vi "Find Button Ering.vi"(4 "Find Ering Setting":T4 {"Options"."Edge Options"."Edge Polarity" items=["All Edges", "Rising Edges", "Falling Edges"]; "Options"."Edge Options"."Minimum Edge Strength" format="%.2f"; "Options"."Edge Options"."Width" step=2; "Options"."Edge Options"."Kernel Size" step=2}, 6 "Find Center Setting":T4 {"Options"."Edge Options"."Edge Polarity" items=["All Edges", "Rising Edges", "Falling Edges"]; "Options"."Edge Options"."Minimum Edge Strength" format="%.2f"; "Options"."Edge Options"."Width" step=2; "Options"."Edge Options"."Kernel Size" step=2}, 7 "Match Position":T7, 8 "error in (no error)":errorcluster, 9 "Ering ROI":T5 {"Contours"."Type" items=["No Selection", "Point", "Line", "Rectangle", "Oval", "Polygon", "Freehand Region", "Annulus", "Unused2", "Unused3", "Broken Line", "Freehand Line", "Rotated Rectangle"]}, 10 "Center ROI":T5 {"Contours"."Type" items=["No Selection", "Point", "Line", "Rectangle", "Oval", "Polygon", "Freehand Region", "Annulus", "Unused2", "Unused3", "Broken Line", "Freehand Line", "Rotated Rectangle"]}, 11 "Image in":T6) -> (0 "error out":errorcluster, 2 "Array of Fittings":T1)   [LabVIEW 2017]
uses:
  <vilib>/vision/Measure.llb/Edge Options.ctl
  <vilib>/vision/Measure.llb/Edge Polarity.ctl
  <vilib>/vision/Image Controls.llb/IMAQ Image.ctl
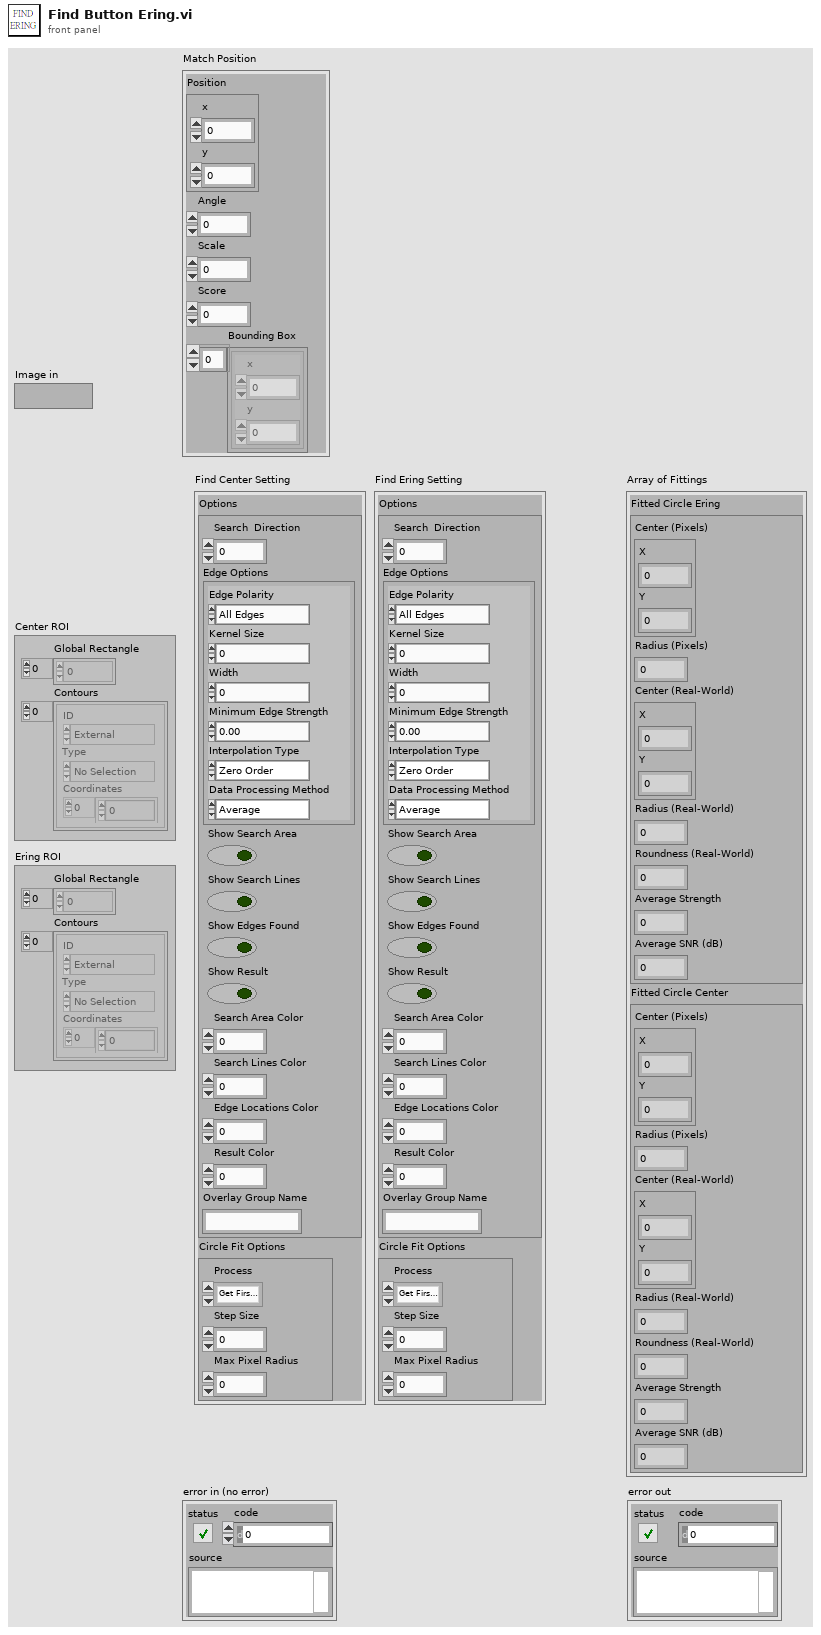
[diagram p1: front panel]
types:
  T1 = cluster{"Fitted Circle Ering":cluster{"Center (Pixels)":cluster{"X":sgl, "Y":sgl}, "Radius (Pixels)":dbl, "Center (Real-World)":cluster{"X":sgl, "Y":sgl}, "Radius (Real-World)":dbl, "Roundness (Real-World)":dbl, "Average Strength":dbl, "Average SNR (dB)":dbl}, "Fitted Circle Center":cluster{"Center (Pixels)":cluster{"X":sgl, "Y":sgl}, "Radius (Pixels)":dbl, "Center (Real-World)":cluster{"X":sgl, "Y":sgl}, "Radius (Real-World)":dbl, "Roundness (Real-World)":dbl, "Average Strength":dbl, "Average SNR (dB)":dbl}}
  T2 = typedef "Edge Options.ctl" = cluster{"Edge Polarity":T3, "Kernel Size":u32, "Width":u32, "Minimum Edge Strength":sgl, "Interpolation Type":enum32{"Zero Order", "Bilinear", "Quadratic", "Cubic", "Bilinear Fixed"}, "Data Processing Method":enum32{"Average", "Median"}}
  T3 = typedef "Edge Polarity.ctl" = u32
  T4 = cluster{"Options":cluster{"Search  Direction":u32, "Edge Options":T2, "Show Search Area":bool, "Show Search Lines":bool, "Show Edges Found":bool, "Show Result":bool, "Search Area Color":u32, "Search Lines Color":u32, "Edge Locations Color":u32, "Result Color":u32, "Overlay Group Name":string}, "Circle Fit Options":cluster{"Process":enum16{"Get First Edge", "Get First + Last Edge", "Get All Edges", "Get Best Edge"}, "Step Size":dbl, "Max Pixel Radius":i32}}
  T5 = typedef "ROI Descriptor" = cluster{"Global Rectangle":i32[], "Contours":cluster{"ID":enum32{"External", "Internal"}, "Type":u32, "Coordinates":i32[]}[]}
  T6 = typedef "IMAQ Image.ctl" = refnum<image>
  T7 = cluster{"Position":cluster{"x":sgl, "y":sgl}, "Angle":sgl, "Scale":sgl, "Score":sgl, "Bounding Box":cluster{"x":sgl, "y":sgl}[]}
  T8 = cluster{"Center (Pixels)":cluster{"X":sgl, "Y":sgl}, "Radius (Pixels)":dbl, "Center (Real-World)":cluster{"X":sgl, "Y":sgl}, "Radius (Real-World)":dbl, "Roundness (Real-World)":dbl, "Average Strength":dbl, "Average SNR (dB)":dbl}
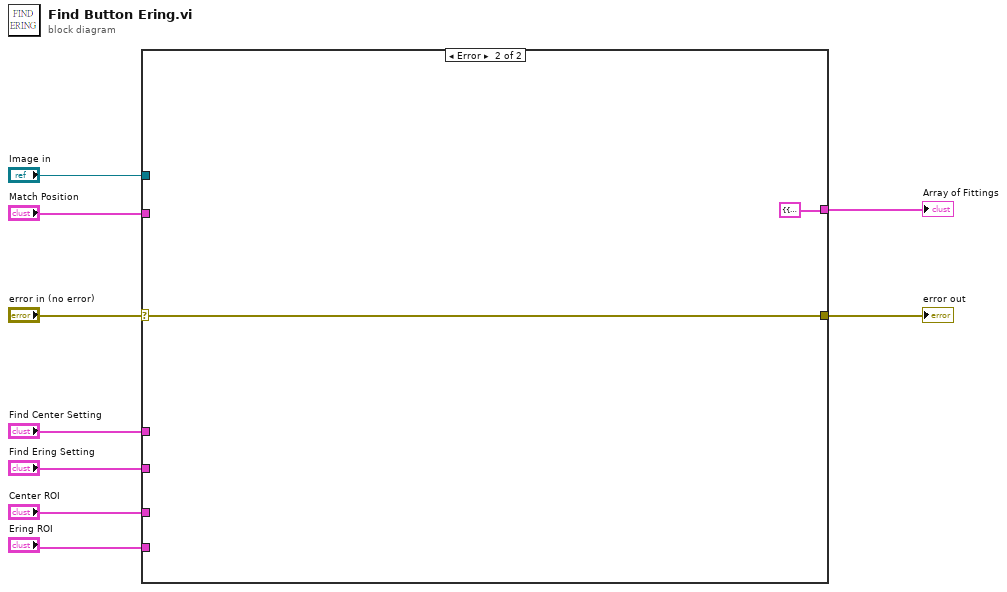
[diagram p0: block diagram]
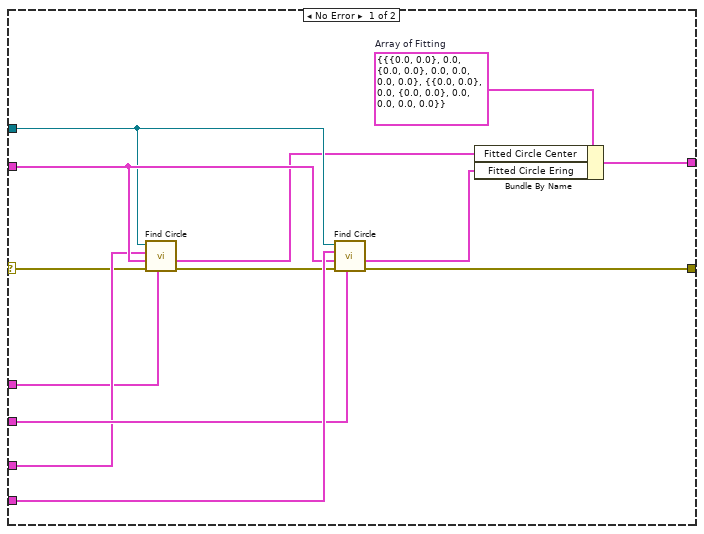
[diagram p2: hidden frame]
diagram:
  n1 = case shown="Error" "error in (no error)" {
    selector: "error in (no error)" -> [w10 w24]
    tunnel: "Ering ROI" -> [w22 _]
    tunnel: "Match Position" -> [w21 _]
    tunnel: "Find Ering Setting" -> [w19 _]
    tunnel: [w18 w24] -> w6
    tunnel: "Image in" -> [w17 _]
    tunnel: "Center ROI" -> [w16 _]
    tunnel: "Find Center Setting" -> [w15 _]
    tunnel: [w11 T1 {"Fitted Circle Ering"={"Center (Pixels)"={"X"=0.0, "Y"=0.0}, "Radius (Pixels)"=0.0, "Center (Real-World)"={"X"=0.0, "Y"=0.0}, "Radius (Real-World)"=0.0, "Roundness (Real-World)"=0.0, "Average Strength"=0.0, "Average SNR (dB)"=0.0}, "Fitted Circle Center"={"Center (Pixels)"={"X"=0.0, "Y"=0.0}, "Radius (Pixels)"=0.0, "Center (Real-World)"={"X"=0.0, "Y"=0.0}, "Radius (Real-World)"=0.0, "Roundness (Real-World)"=0.0, "Average Strength"=0.0, "Average SNR (dB)"=0.0}} ("Array of Fitting")] -> w2
    frame No Error {
      w14 = T1 {"Fitted Circle Ering"={"Center (Pixels)"={"X"=0.0, "Y"=0.0}, "Radius (Pixels)"=0.0, "Center (Real-World)"={"X"=0.0, "Y"=0.0}, "Radius (Real-World)"=0.0, "Roundness (Real-World)"=0.0, "Average Strength"=0.0, "Average SNR (dB)"=0.0}, "Fitted Circle Center"={"Center (Pixels)"={"X"=0.0, "Y"=0.0}, "Radius (Pixels)"=0.0, "Center (Real-World)"={"X"=0.0, "Y"=0.0}, "Radius (Real-World)"=0.0, "Roundness (Real-World)"=0.0, "Average Strength"=0.0, "Average SNR (dB)"=0.0}}  # Array of Fitting
      n2 = call "Find Circle.vi"("Find Circle Setting"=w15, "error in (no error)"=w10, "Matches (pixel)"=w21, "ROI Descriptor"=w16, "Image"=w17) -> ("error out"=w20:errorcluster, "Fitted Circle"=w12:T8)  [unwired: 3 in, 2 out]
      n3 = call "Find Circle.vi"("Find Circle Setting"=w19, "error in (no error)"=w20, "Matches (pixel)"=w21, "ROI Descriptor"=w22, "Image"=w17) -> ("error out"=w18:errorcluster, "Fitted Circle"=w13:T8)  [unwired: 3 in, 2 out]
      n4 = Bundle By Name(cluster=w14, "Fitted Circle Center"=w12, "Fitted Circle Ering"=w13) -> (w11:T1)
    }
    frame Error {
    }
  }
  "error out" <- w6
  "Array of Fittings" <- w2
